vi "avoid_double_click_event_struct.vi"() -> ()   [LabVIEW 2013]
panel:
  in  "disable time":u32
  out "Zeit":string
  in  "wie kurz":u32
  in  "wie lange":u32
  out "bool kurz":bool
  out "bool lange":bool
  in  "Kurz":bool
  in  "Lange":bool
  in  "Stopp":bool
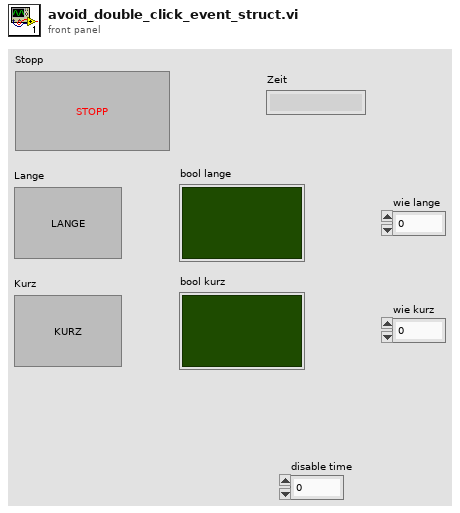
[diagram p1: front panel]
types:
  T1 = enum8{"Enabled", "Disabled", "Disabled and Grayed Out"}
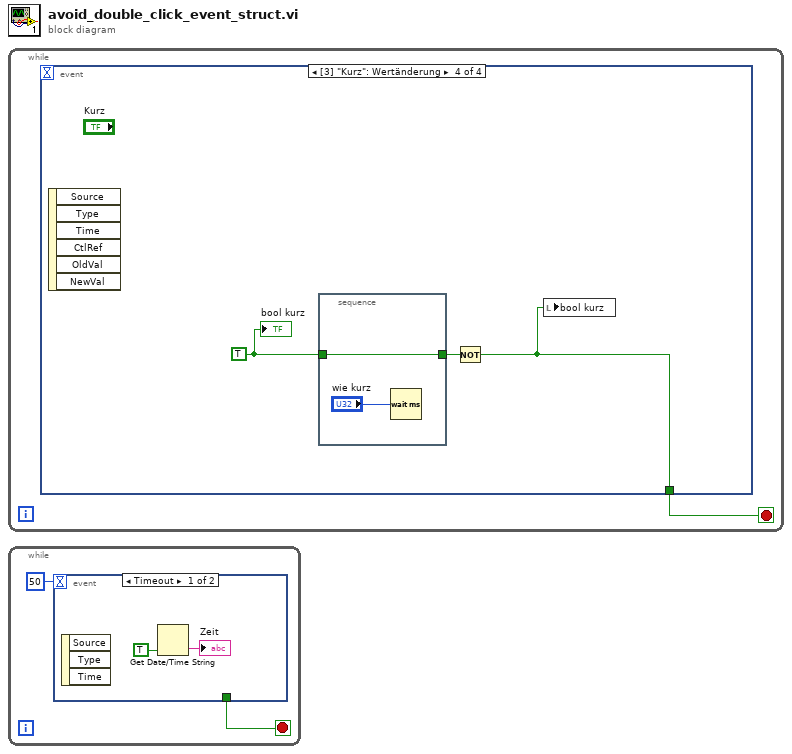
[diagram p0: block diagram]
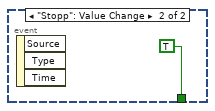
[diagram p2: hidden frame]
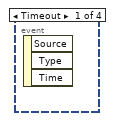
[diagram p3: hidden frame]
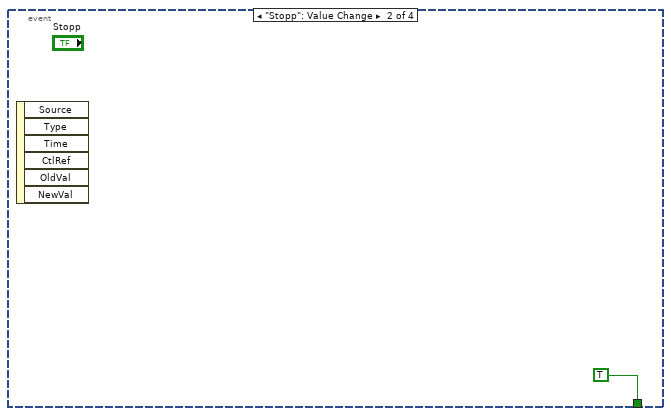
[diagram p4: hidden frame]
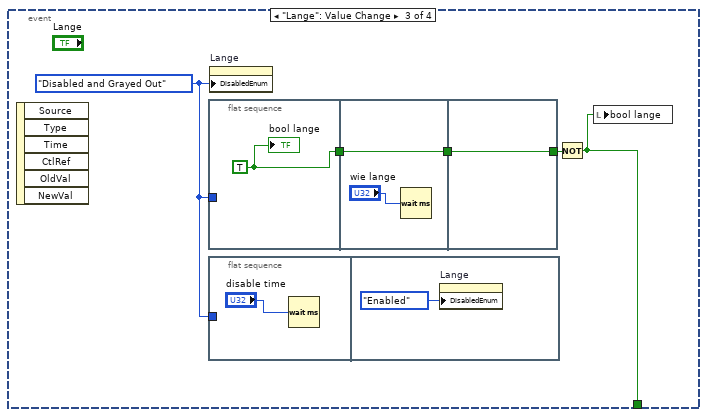
[diagram p5: hidden frame]
diagram:
  n1 = while {
    stop <- w1 stop-if-true
    n2 = event shown="[3] \"Kurz\": Wertänderung" {
      selector: _ -> [_ _ _ _]
      dyn-events: _ -> [_ _ _ _]
      timeout: _ -> [_ _ _ _]
      tunnel: [_ TRUE w6 w14] -> w1
      event Timeout {
        n3 = event-data() -> ()  [unwired: 1 in, 3 out]
      }
      event "Stopp": Value Change {
        n4 = event-data() -> ()  [unwired: 1 in, 6 out]
      }
      event "Lange": Value Change {
        w3 = T1."Disabled and Grayed Out" ("Deaktiviert")
        n5 = event-data() -> ()  [unwired: 1 in, 6 out]
        n6 = flat-sequence {
          tunnel: [w10] -> w5
          tunnel: w3 -> [_]
          tunnel: w5 -> [w11]
          tunnel: [w11] -> w4
          tunnel: [w13] -> w7
          tunnel: w4 -> [w13]
          frame #0 {
            w10 = TRUE
            "bool lange" <- w10
          }
          frame #1 {
            n7 = Wait (ms)(milliseconds to wait="wie lange") -> ()  [unwired: 1 out]
          }
          frame #2 {
          }
        }
        n8 = flat-sequence {
          tunnel: w3 -> [_]
          frame #0 {
            n9 = Wait (ms)(milliseconds to wait="disable time") -> ()  [unwired: 1 out]
          }
          frame #1 {
            n10 = property on="Lange" class="Bool."("DisabledEnum"=T1."Enabled" ("Deaktiviert")) -> ()  [unwired: 2 in, 2 out]
          }
        }
        n11 = property on="Lange" class="Bool."("DisabledEnum"=w3) -> ()  [unwired: 2 in, 2 out]
        n12 = Not(x=w7) -> (.not. x?=w6:bool)
        n13 = local write "bool lange"(w6) -> ()
      }
      event "Kurz": Value Change {
        w16 = TRUE
        n14 = event-data() -> ()  [unwired: 1 in, 6 out]
        n15 = stacked-sequence {
          tunnel: w16 -> [w18]
          tunnel: [w18] -> w15
          frame #0 {
            n16 = Wait (ms)(milliseconds to wait="wie kurz") -> ()  [unwired: 1 out]
          }
        }
        n17 = Not(x=w15) -> (.not. x?=w14:bool)
        n18 = local write "bool kurz"(w14) -> ()
        "bool kurz" <- w16
      }
    }
  }
  n19 = while {
    stop <- w20 stop-if-true
    n20 = event shown="[0] Timeout" {
      selector: _ -> [_ _]
      dyn-events: _ -> [_ _]
      timeout: 50 -> [_ _]
      tunnel: [_ TRUE] -> w20
      event Timeout {
        n21 = event-data() -> ()  [unwired: 1 in, 3 out]
        n22 = Get Date/Time String(want seconds? (F)=TRUE ("Angabe von Sekunden? (F)")) -> (time string=→"Zeit":string)  [unwired: 2 in, 1 out]
      }
      event "Stopp": Value Change {
        n23 = event-data() -> ()  [unwired: 1 in, 3 out]
      }
    }
  }
